vi "PacketToState.vi"(6 "MarkerIdx":i32=1, 7 "DataPacket":string, 9 "DistanceThresh":sgl=0.001, 11 "BodyIdx":i32) -> (2 "Sync":bool, 3 "State":dbl[](array[numeric]))   [LabVIEW 2011]
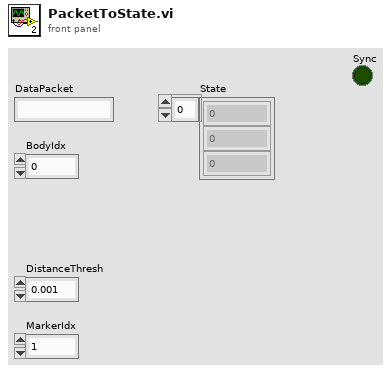
[diagram p1: front panel]
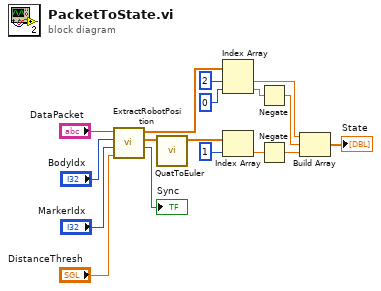
[diagram p0: block diagram]
diagram:
  n1 = call "ExtractRobotPosition.vi"("DistanceThresh"="DistanceThresh", "MarkerIdx"="MarkerIdx", "BodyIdx"="BodyIdx", "Data"="DataPacket") -> ("Found?"=→"Sync":bool, "RigidBodyOri"=w13:sgl[], "RigidBodyPos"=w1:sgl[])  [unwired: 5 in]
  n2 = call "QuatToEuler.vi"("RigidBodyOri"=w13) -> ("Array"=w5:sgl[])  [unwired: 10 in]
  n3 = Index Array(array=w1, index #1=2 ("index"), index #2=0 ("index")) -> (element #1=w15:sgl, element #2=w12:sgl)
  n4 = Index Array(array=w5, index=1) -> (element=w17:sgl)
  n5 = Negate(x=w12) -> (-x=w16:sgl)
  n6 = Negate(x=w17) -> (-x=w4:sgl)
  n7 = Build Array(w15, w16, w4) -> (→"State":sgl[])
